vi "wotw.vi"() -> ()   [LabVIEW 2021]
panel:
  out "Numeric":dbl
  out "Boolean 2":bool
  out "Boolean":bool
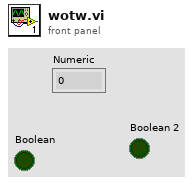
[diagram p1: front panel]
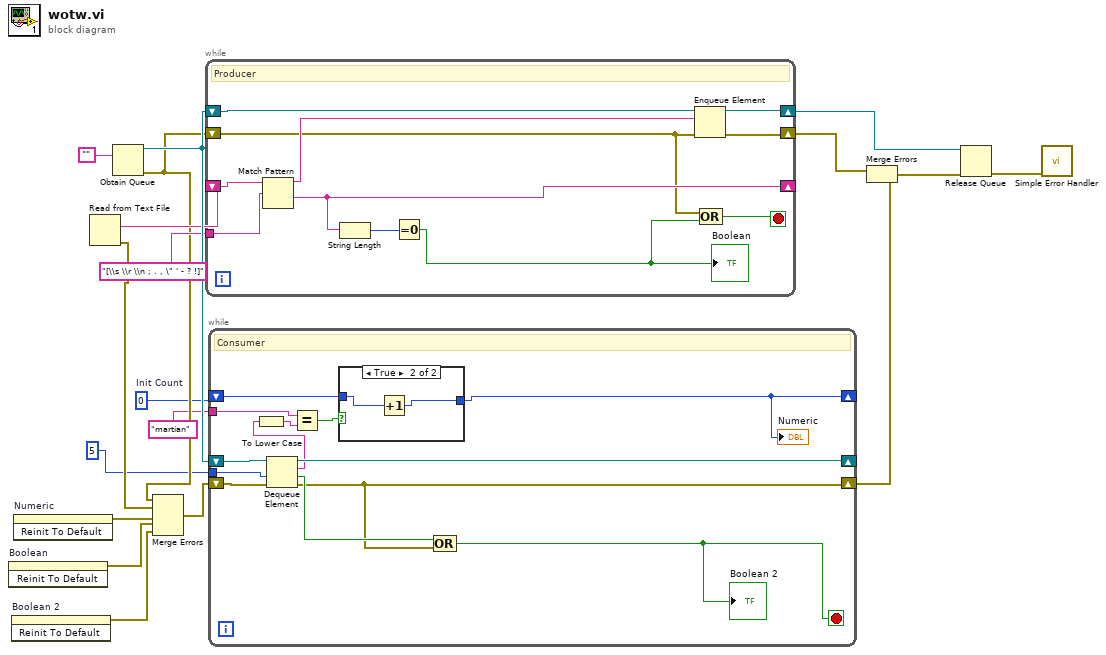
[diagram p0: block diagram]
diagram:
  w3 = 0  # Init Count
  n1 = invoke on="Boolean" class="Bool (strict)" method="Reinit To Default"() -> (error out=w5:errorcluster)  [unwired: 3 in, 2 out]
  n2 = invoke on="Boolean 2" class="Bool (strict)" method="Reinit To Default"() -> (error out=w4:errorcluster)  [unwired: 3 in, 2 out]
  n3 = invoke on="Numeric" class="DigNum (strict)" method="Reinit To Default"() -> (error out=w6:errorcluster)  [unwired: 3 in, 2 out]
  n4 = Read from Text File() -> (text=w11:string, error out=w8:errorcluster)  [unwired: 4 in, 2 out]
  n5 = Obtain Queue(element data type="") -> (queue out=w15:refnum<queue>, error out=w9:errorcluster)  [unwired: 4 in, 1 out]
  n6 = Merge Errors(w9, w8, w6, w5, w4) -> (w7:errorcluster)
  n7 = while {
    shift-right: [w28] -> w17
    shift-left: w15 -> [w29]
    shift-right: [w27] -> w13
    shift-left: w9 -> [w20]
    shift-right: [w22] -> _
    shift-left: w11 -> [w26]
    tunnel: "[\\s \\r \\n ; . , \" ' - ? !]" -> [w24]
    stop <- w21 stop-if-true
    # "Producer"
    n8 = Match Pattern(string=w26, regular expression=w24) -> (before substring=w25:string, after substring=w22:string)  [unwired: 1 in, 2 out]
    n9 = String Length(string=w22) -> (length=w23:i32)
    n10 = Equal To 0?(x=w23) -> (x = 0?=w19:bool)
    "Boolean" <- w19
    n11 = Enqueue Element(queue=w29, element=w25, error in (no error)=w20) -> (queue out=w28:refnum<queue>, error out=w27:errorcluster)  [unwired: 1 in, 1 out]
    n12 = Compound Arithmetic op=OR(w20, w19) -> (w21:bool)
  }
  n13 = while {
    shift-right: [w40] -> _
    shift-left: w15 -> [w41]
    shift-right: [w33] -> w14
    shift-left: w7 -> [w42]
    shift-right: [w30] -> _
    shift-left: w3 -> [w39]
    tunnel: "martian" -> [w38]
    tunnel: 5 -> [w32]
    stop <- w31 stop-if-true
    # "Consumer"
    n14 = Dequeue Element(queue=w41, timeout in ms (-1)=w32, error in (no error)=w42) -> (queue out=w40:refnum<queue>, element=w36:string, timed out?=w34:bool, error out=w33:errorcluster)
    n15 = To Lower Case(string=w36) -> (all lower case string=w37:string)
    n16 = Equal?(x=w38, y=w37) -> (x = y?=w35:bool)
    n17 = case shown="True" w35 {
      tunnel: w39 -> [w43 w45]
      tunnel: [w43 w44] -> w30
      frame False {
      }
      frame True {
        n18 = Increment(x=w45) -> (x+1=w44:i32)
      }
    }
    "Numeric" <- w30
    n19 = Compound Arithmetic op=OR(w34, w33) -> (w31:bool)
    "Boolean 2" <- w31
  }
  n20 = Merge Errors(w13, w14) -> (w12:errorcluster)
  n21 = Release Queue(queue=w17, error in (no error)=w12) -> (error out=w16:errorcluster)  [unwired: 1 in, 2 out]
  n22 = call <vilib>:"Simple Error Handler.vi"("error in (no error)"=w16) -> ()  [unwired: 4 in, 5 out]
